vi "Simple_SMT_IQ_Spectrum.vi"() -> ()   [LabVIEW 2014]
uses:
  <vilib>/addons/Spectral Measurements Toolset/LVSupport/SMT BZ spectrum settings.ctl
  <instrlib>/niRFSA/niRFSA.llb/niRFSA Acquisition Types.ctl
  <instrlib>/niRFSA/niRFSA.llb/niRFSA Trigger Terminals.ctl
  <instrlib>/niRFSA/niRFSA.llb/niRFSA Trigger DigEdge - Edge Values.ctl
  <vilib>/measure/masml.llb/ma_sml_Averaging Parameters.ctl
  <vilib>/measure/masml.llb/ma_sml_Averaging Settings.ctl
  <instrlib>/niRFSA/niRFSA.llb/niRFSA Configure Digital Edge Ref Trigger.vi
  <instrlib>/niRFSA/niRFSA.llb/niRFSA Fetch IQ (Complex Cluster 1Rec 1Chan).vi
  <instrlib>/niRFSA/niRFSA.llb/niRFSA Get IQ Components (Complex Cluster).vi
  <vilib>/addons/Spectral Measurements Toolset/LVSupport/SMT Zoom Power Spectrum (Complex Input).vi
  <vilib>/measure/NI_MAPro.lvlib
  <vilib>/addons/Spectral Measurements Toolset/niSMT.lvlib
panel:
  out "Acquisition:IQ:IQ Rate (S/s)":dbl
  out "x-y":dbl
  in  "Configure Spectrum Settings":T1={"center frequency"=1000000000.0, "span"=-1.0, "resolution bandwidth"=-1.0} {"resolution bandwidth" format="%.2p"; "center frequency" format="%.2p"; "span" format="%.2p"}
  in  "advanced settings":T2={"window"=enum."Flat Top", "spectral lines"=-1, "effective band specification"={"fl"=0.0, "fh"=0.5}, "RBW definition"=enum."3dB"} {"effective band specification"."fh" format="%.2f"; "effective band specification"."fl" format="%.2f"}
  in  "Samples per fetch":i32=10000
  in  "stop":bool
  in  "Tab Control":enum32{"I Data", "Q Data", "Zoom Spectrum"}(tab)=enum."Zoom Spectrum"
  out "I Data":cluster{"t0":dbl, "dt":dbl, "Y":dbl[]}(graph)
  out "Q Data":cluster{"t0":dbl, "dt":dbl, "Y":dbl[]}(graph)
  out "Waveform Graph":cluster{"f0":dbl, "df":dbl, "spectrum":dbl[]}(graph)
  in  "Unit conversion settings":T3={"units"=enum."dBm", "peak scaling"=enum."rms", "psd?"=FALSE, "impedance(ohm)"=50.0} {"impedance(ohm)" format="%.2f"}
  in  "IQ rate (S/s)":dbl=1000000.0 format="%#_6p"
  in  "Reference level (dBm)":dbl format="%.2f"
  in  "Resource name":refnum<k15>="5600"
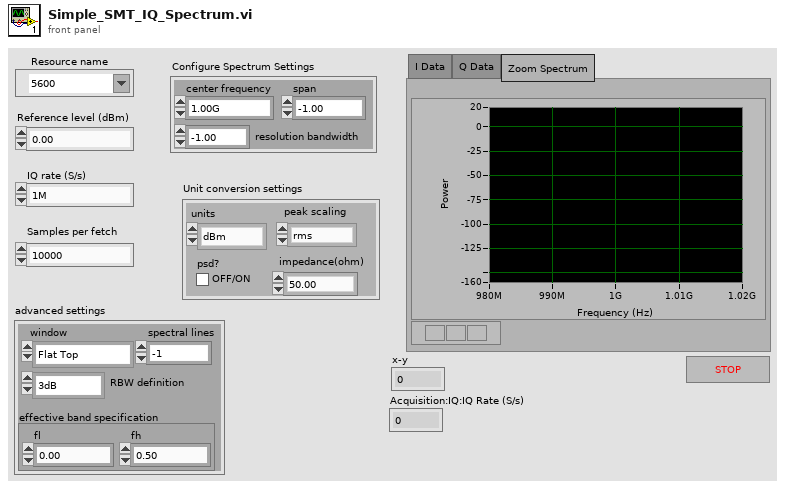
[diagram p1: front panel]
types:
  T1 = typedef "niSMT.lvlib/SMT BZ spectrum settings.ctl" = cluster{"center frequency":dbl, "span":dbl, "resolution bandwidth":dbl}
  T2 = cluster{"window":enum16{"None ", "Hanning", "Hamming", "Blackman-Harris", "Exact Blackman", "Blackman", "Flat Top", "4 Term B-Harris ", "7 Term B-Harris", "Low Sidelobe"}, "spectral lines":i32, "effective band specification":cluster{"fl":dbl, "fh":dbl}, "RBW definition":enum16{"3dB", "6dB", "ENBW", "bin width"}}
  T3 = cluster{"units":enum16{"V", "V^2", "W", "dBm", "dBW", "dBV", "dBmV", "dBuV"}, "peak scaling":enum16{"rms", "pk"}, "psd?":bool, "impedance(ohm)":dbl}
  T4 = typedef "niRFSA Trigger DigEdge - Edge Values.ctl" = i32
  T5 = typedef "niRFSA Trigger Terminals.ctl" = string
  T6 = typedef "niRFSA Acquisition Types.ctl" = i32
  T7 = cluster{"type":enum16{"real", "complex modulated"}, "IQ Carrier Frequency":dbl}
  T8 = typedef "niSMT.lvlib/SMT zoom settings.ctl" = cluster{"zoom FFT settings":T9, "frequency shift":dbl, "data format":enum16{"real", "complex modulated (array)", "complex modulated (interleaved)"}}
  T9 = typedef "NI_MAPro.lvlib/ma_sml_ND Zoom FFT Settings.ctl" = cluster{"zoom settings":cluster{"center frequency":dbl, "zoom":i32, "trim":dbl}, "FFT settings":cluster{"window":u16, "FFT size":i32}}
  T10 = enum16{"no averaging", "vector averaging", "RMS averaging", "peak hold"}
  T11 = typedef "NI_MAPro.lvlib/ma_sml_Averaging Parameters.ctl" = cluster{"averaging type":enum16{"no averaging", "vector averaging", "RMS averaging", "peak hold"}, "averaging settings":T12}
  T12 = typedef "NI_MAPro.lvlib/ma_sml_Averaging Settings.ctl" = cluster{"weighting type":enum16{"linear", "exponential"}, "weighting settings":cluster{"size":dbl, "linear weighting mode":enum16{"one shot", "auto restart one shot", "moving average", "continuous"}}}
  T13 = typedef "NI_MAPro.lvlib/ma_sml_Spectral Info.ctl" = cluster{"spectrum type":enum16{"FFT Spectrum [complex]", "Amplitude [Magnitude]", "Power [Magnitude^2]", "Cross Spectrum [complex]", "Frequency Response [Complex]"}, "linear/dB":enum16{"linear", "dB"}, "window":u16, "window size":i32, "FFT size":i32}
  T14 = typedef "NI_MAPro.lvlib/ma_sml_Spectrum Cluster (real).ctl" = cluster{"f0":dbl, "df":dbl, "spectrum":dbl[]}
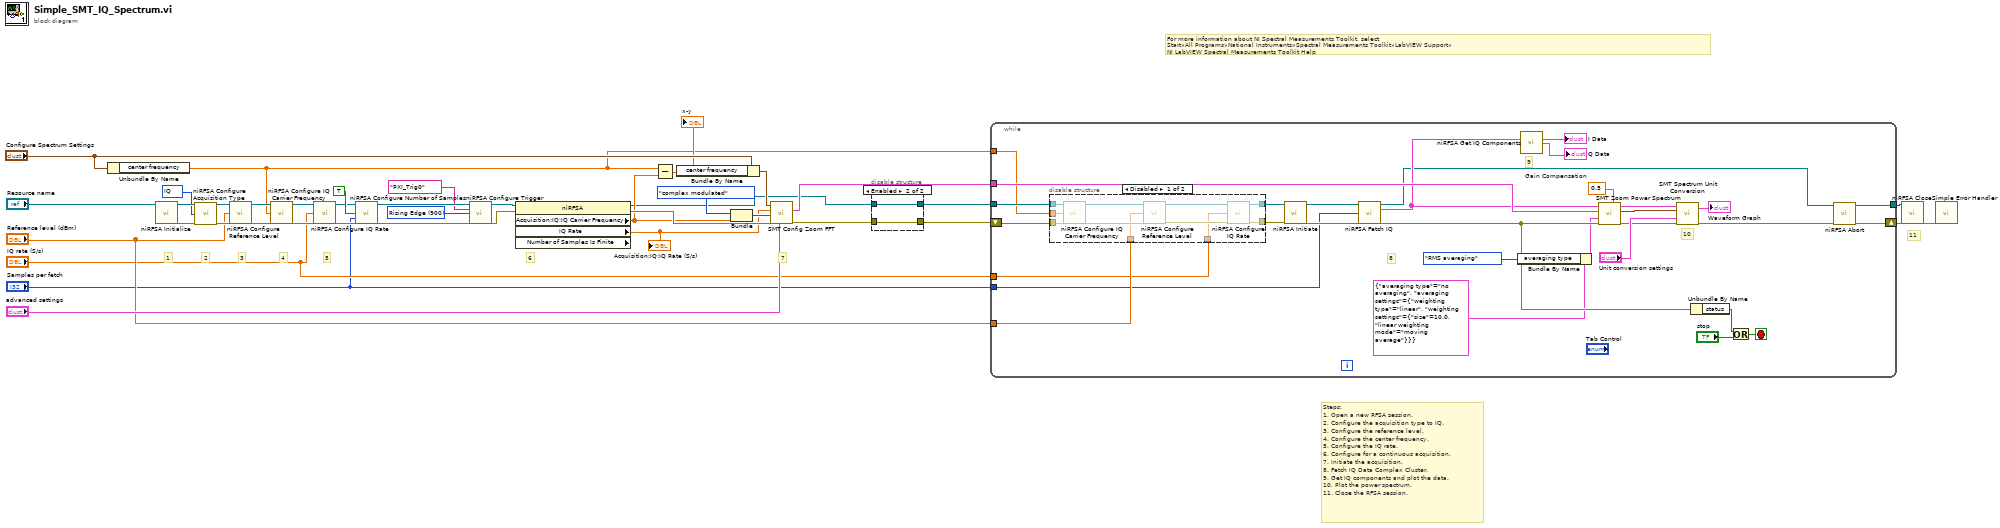
[diagram p0: block diagram]
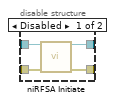
[diagram p2: hidden frame]
diagram:
  w6 = T4 900 items=["Rising Edge"=900, "Falling Edge"=901] ("edge")
  w31 = T6 100 items=["IQ"=100, "Spectrum"=101] ("acquisition type")
  # "For more information about NI Spectral Measurements Toolkit, select \nStart»All Programs»National Instruments»Spectral Measurements Toolkit»LabVIEW Support»\nNI LabVIEW Spectral Measurements Toolkit Help"
  # "11"
  # "7"
  # "6"
  # "5"
  # "4"
  # "3"
  # "2"
  # "1"
  # "Steps:\n1. Open a new RFSA session.\n2. Configure the acquisition type to IQ.\n3. Configure the reference level.\n4. Configure the center frequency.\n5. Configure the IQ rate.\n6. Configure for a continuous acquisition.\n7. Initiate the acquisition.\n8. Fetch IQ Data Complex Cluster.\n9. Get IQ components and plot the data.\n10. Plot the power spectrum.\n11. Close the RFSA session."
  n1 = Unbundle By Name("Configure Spectrum Settings") -> ("center frequency"=w10:dbl)
  n2 = call <instrlib>:"niRFSA Initialize.vi"("resource name"="Resource name") -> ("instrument handle"=w34:refnum<k15>, "error out"=w35:errorcluster)  [unwired: 4 in, 9 out]
  n3 = call <instrlib>:"niRFSA Configure Acquisition Type.vi"("instrument handle"=w34, "acquisition type"=w31, "error in"=w35) -> ("instrument handle out"=w37:refnum<k15>, "error out"=w36:errorcluster)  [unwired: 1 in, 10 out]
  n4 = call <instrlib>:"niRFSA Configure Reference Level.vi"("instrument handle"=w37, "reference level (dBm)"="Reference level (dBm)", "error in"=w36) -> ("instrument handle out"=w26:refnum<k15>, "error out"=w23:errorcluster)  [unwired: 1 in, 10 out]
  n5 = call <instrlib>:"niRFSA Configure IQ Carrier Frequency.vi"("instrument handle"=w26, "carrier frequency"=w10, "error in"=w23) -> ("instrument handle out"=w25:refnum<k15>, "error out"=w24:errorcluster)  [unwired: 11 out]
  n6 = call <instrlib>:"niRFSA Configure IQ Rate.vi"("instrument handle"=w25, "IQ rate (S/s)"="IQ rate (S/s)", "error in"=w24) -> ("instrument handle out"=w28:refnum<k15>, "error out"=w29:errorcluster)  [unwired: 1 in, 10 out]
  n7 = call <instrlib>:"niRFSA Configure Number of Samples.vi"("instrument handle"=w28, "number of samples is finite"=TRUE, "samples per record"="Samples per fetch", "error in"=w29) -> ("instrument handle out"=w14:refnum<k15>, "error out"=w13:errorcluster)  [unwired: 1 in, 9 out]
  n8 = call-poly <instrlib>:"niRFSA Configure Trigger.vi"("instrument handle"=w14, "source"=T5 "PXI_Trig0", "edge"=w6, "error in"=w13) -> ("instrument handle out"=w12:refnum<k15>, "error out"=w11:errorcluster)  [unwired: 10 in]
  n9 = property class="niRFSA" props=["Acquisition:IQ:IQ Carrier Frequency", "IQ Rate", "Number of Samples Is Finite"](reference=w12, error in=w11) -> (reference out=w5:refnum<k15>, error out=w40:errorcluster, "Acquisition:IQ:IQ Carrier Frequency"=w15:dbl, "IQ Rate"=w19:dbl)  [unwired: 1 out]
  "Acquisition:IQ:IQ Rate (S/s)" <- w19
  n10 = Subtract(x=w10, y=w15) -> (x-y=w16:dbl)
  "x-y" <- w16
  n11 = Bundle By Name(cluster="Configure Spectrum Settings", "center frequency"=w16) -> (w17:T1)
  n12 = Bundle("type"=enum16{"real", "complex modulated"}."complex modulated", "IQ Carrier Frequency"=w15) -> (w22:T7)  [unwired: 1 out]
  n13 = call <vilib>:"SMT Config Zoom FFT.vi"("advanced settings"="advanced settings", "error in (no error)"=w40, "input signal settings"=w22, "fs"=w19, "spectrum settings"=w17) -> ("error out"=w4:errorcluster, "SMT zoom settings"=w21:T8)  [unwired: 5 out]
  n14 = disable-structure shown="Enabled" {
    disable-tunnel: w5 -> [w44 w46]
    disable-tunnel: w4 -> [w43 w45]
    disable-tunnel: [w42 w45] -> w3
    disable-tunnel: [w41 w46] -> w2
    frame Disabled {
      n15 = call <instrlib>:"niRFSA Initiate.vi"("instrument handle"=w44, "error in"=w43) -> ("instrument handle out"=w41:refnum<k15>, "error out"=w42:errorcluster)  [unwired: 12 out]
    }
    frame Enabled {
    }
  }
  n16 = while {
    shift-right: [w49] -> w38
    shift-left: w3 -> [w58]
    tunnel: [w50] -> w32
    tunnel: w21 -> [w71]
    tunnel: "Samples per fetch" -> [w47]
    tunnel: w2 -> [w57]
    tunnel: w10 -> [w56]
    tunnel: "Reference level (dBm)" -> [w55]
    tunnel: "IQ rate (S/s)" -> [w54]
    stop <- w75 stop-if-true
    w66 = 0.5  # Gain Compensation
    # "10"
    # "9"
    # "8"
    n17 = disable-structure shown="Disabled" {
      disable-tunnel: w58 -> [w88 w89]
      disable-tunnel: w57 -> [w87 w90]
      disable-tunnel: w56 -> [w86 _]
      disable-tunnel: w55 -> [w83 _]
      disable-tunnel: w54 -> [w80 _]
      disable-tunnel: [w79 w90] -> w53
      disable-tunnel: [w78 w89] -> w52
      frame Disabled {
        n18 = call <instrlib>:"niRFSA Configure IQ Carrier Frequency.vi"("instrument handle"=w87, "carrier frequency"=w86, "error in"=w88) -> ("instrument handle out"=w85:refnum<k15>, "error out"=w84:errorcluster)  [unwired: 11 out]
        n19 = call <instrlib>:"niRFSA Configure Reference Level.vi"("instrument handle"=w85, "reference level (dBm)"=w83, "error in"=w84) -> ("instrument handle out"=w82:refnum<k15>, "error out"=w81:errorcluster)  [unwired: 1 in, 10 out]
        n20 = call <instrlib>:"niRFSA Configure IQ Rate.vi"("instrument handle"=w82, "IQ rate (S/s)"=w80, "error in"=w81) -> ("instrument handle out"=w79:refnum<k15>, "error out"=w78:errorcluster)  [unwired: 1 in, 10 out]
      }
      frame Enabled {
      }
    }
    n21 = call <instrlib>:"niRFSA Initiate.vi"("instrument handle"=w53, "error in"=w52) -> ("instrument handle out"=w60:refnum<k15>, "error out"=w59:errorcluster)  [unwired: 12 out]
    n22 = call-poly <instrlib>:"niRFSA Fetch IQ.vi"("instrument handle"=w60, "samples to read (-1)"=w47, "error in"=w59) -> ("instrument handle out"=w48:refnum<k15>, "data"=w70:cluster{"t0":dbl, "dt":dbl, "Y":cdb[]}, "error out"=w72:errorcluster)  [unwired: 2 in, 8 out]
    n23 = Bundle By Name(cluster=T11 {"averaging type"=enum."no averaging", "averaging settings"={"weighting type"=enum."linear", "weighting settings"={"size"=10.0, "linear weighting mode"=enum."moving average"}}} ("averaging parameters"), "averaging type"=T10."RMS averaging") -> (w61:T11)
    n24 = call-poly <instrlib>:"niRFSA Get IQ Components.vi"("data"=w70) -> ("I"=→"I Data":cluster{"t0":dbl, "dt":dbl, "Y":dbl[]}, "Q"=→"Q Data":cluster{"t0":dbl, "dt":dbl, "Y":dbl[]})  [unwired: 1 in, 12 out]
    n25 = call-poly <vilib>:"SMT Zoom Power Spectrum.vi"("gain compensation"=w66, "error in (no error)"=w72, "averaging parameters"=w61, "SMT zoom settings"=w71, "signal in"=w70) -> ("error out"=w69:errorcluster, "spectral info"=w68:T13, "power spectrum"=w67:T14)  [unwired: 1 in, 3 out]
    n26 = call <vilib>:"SMT Spectrum Unit Conversion.vi"("error in (no error)"=w69, "unit conversion settings"="Unit conversion settings", "spectral info in"=w68, "power spectrum"=w67) -> ("error out"=w51:errorcluster, "unit converted spectrum"=→"Waveform Graph":cluster{"f0":dbl, "df":dbl, "spectrum":dbl[]})  [unwired: 6 out]
    n27 = Unbundle By Name(w72) -> ("status"=w77:bool)
    n28 = Or(x=w77, y="stop") -> (x .or. y?=w75:bool)
    n29 = call <instrlib>:"niRFSA Abort.vi"("instrument handle"=w48, "error in"=w51) -> ("instrument handle out"=w50:refnum<k15>, "error out"=w49:errorcluster)  [unwired: 12 in]
  }
  n30 = call <instrlib>:"niRFSA Close.vi"("instrument handle"=w32, "error in"=w38) -> ("error out"=w33:errorcluster)  [unwired: 13 out]
  n31 = call <vilib>:"Simple Error Handler.vi"("error in (no error)"=w33) -> ()  [unwired: 1 in, 8 out]
